vi "Autonomous Independent.vi"() -> ()   [LabVIEW 2019]
doc: "This VI is called when autonomous begins, and will automatically be terminated when autonomous ends. You can carry out timed or sensor driven robot movement independently without needing to return to the caller."
uses:
  Globals/Drive_Globals.vi
  Globals/Turret_Globals.vi
  Subsystems/Turret/Turret_States.ctl
  Subsystems/Turret/Turret_Cluster.ctl
  Globals/Flywheel_Globals.vi
  Subsystems/Flywheel/Flywheel_States.ctl
  Subsystems/Flywheel/Flywheel_Cluster.ctl
  Subsystems/Magazine/Magazine_States.ctl
  Subsystems/Magazine/Magazine_Cluster.ctl
  Globals/Magazine_Globals.vi
  Subsystems/Drive/Drive_States.ctl
  Subsystems/Drive/Drive_Cluster.ctl
  Subsystems/Intake/Intake_States.ctl
  Subsystems/Intake/Intake_Cluster.ctl
  Globals/Intake_Globals.vi
  Globals/Dash_Globals.vi
panel:
  out "Name of Play":string
  # "e"
  # "Be sure to right-click and choose Data Operations>>Make Current Value default if you want to save the array values with the VI"
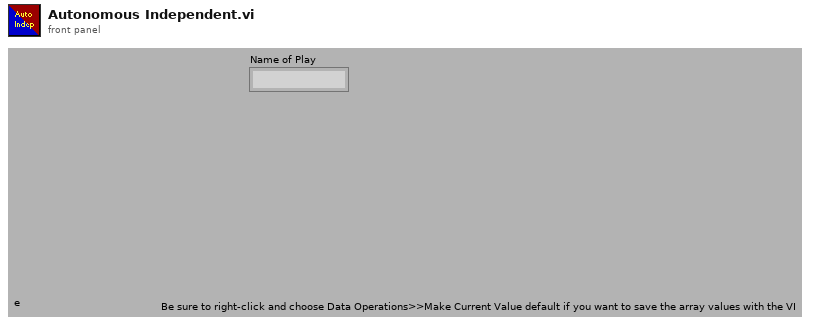
[diagram p1: front panel]
types:
  T1 = typedef "CTRE_PigeonIMU_DeviceRef.ctl" = cluster{"DeviceStatus":errorcluster, "Device Number":u8, "Type":T2, "Device ID":u32, "Handle":u64, "UsageFrame":u32, "Library Path":path}
  T2 = typedef "CTRE_PigeonIMU_ConnectionType.ctl" = u32
  T3 = typedef "WPI_MotorControlDeviceRef.ctl" = cluster{"DeviceStatus":errorcluster, "Type":T4, "PWM":cluster{"PWM Channel":T5, "DeadBand":T6}, "CAN":cluster{"Device Number":u8, "SetOutput VI Ref":variant, "GetOutput VI Ref":variant, "Enable VI Ref":variant, "Disable VI Ref":variant, "Data":variant}, "Invert":bool, "DIO PWM":cluster{"PWM \"Enable\" Channel":T5, "DIOChannel":T7, "PWM Rate":dbl}}
  T4 = typedef "WPI_MotorControlType.ctl" = enum16{"PWM", "CAN", "DIO PWM"}
  T5 = typedef "FPGA_DIOPWMChannel.ctl" = enum8{"PWM 0", "PWM 1", "PWM 2", "PWM 3", "PWM 4", "PWM 5", "PWM 6", "PWM 7", "PWM 8", "PWM 9", "PWM MXP 0", "PWM MXP 1", "PWM MXP 2", "PWM MXP 3", "PWM MXP 4", "PWM MXP 5", "PWM MXP 6", "PWM MXP 7", "PWM MXP 8", "PWM MXP 9", "Invalid"}
  T6 = typedef "WPI_PWMDeadband.ctl" = cluster{"Name":string, "maxPositivePwm":i32, "minPositivePwm":i32, "centerPwm":i32, "maxNegativePwm":i32, "minNegativePwm":i32, "angularRange":u16}
  T7 = typedef "FPGA_DIOChannel.ctl" = enum8{"DIO 0", "DIO 1", "DIO 2", "DIO 3", "DIO 4", "DIO 5", "DIO 6", "DIO 7", "DIO 8", "DIO 9", "DIO MXP 0", "DIO MXP 1", "DIO MXP 2", "DIO MXP 3", "DIO MXP 4", "DIO MXP 5", "DIO MXP 6", "DIO MXP 7", "DIO MXP 8", "DIO MXP 9", "DIO MXP 10", "DIO MXP 11", "DIO MXP 12", "DIO MXP 13", "DIO MXP 14", "DIO MXP 15", "SPI Port CS1", "SPI Port CS2", "SPI Port CS3", "SPI Port MISO", "SPI Port MOSI", "Invalid"}
  T8 = typedef "Flywheel_Cluster.ctl" = cluster{"Flywheel_Throttle":dbl, "Control_States":T9, "Auto_Speed":bool, "Flywheel_On":bool, "Parameter_1":dbl, "Parameter_2":dbl, "Auto_Notifier":refnum<notifier>, "Step":dbl}
  T9 = typedef "Flywheel_States.ctl" = enum16{"No-Op", "Percent_Voltage", "Speed_Control_Manual", "Speed_Control_Auto", "Command_SpinUp", "Command_SpinUpAuto"}
  T10 = typedef "Turret_Cluster.ctl" = cluster{"Auto-Target?":bool, "Control_State":T11, "Turret_Spin_Speed":dbl, "Turret_Spin_Speed_Control?":bool, "Step":dbl, "Parameter_1":dbl, "Parameter_2":dbl, "Parameter_3":dbl, "Auto_Notifier":refnum<notifier>, "GoToZero?":bool}
  T11 = typedef "Turret_States.ctl" = enum16{"Manual_Percent_Voltage", "Manual_Speed_Control", "Auto-Target", "Command_TurnToPosition", "Command_Auto_Target", "GoToZero"}
  T12 = typedef "Magazine_Cluster.ctl" = cluster{"Fire":bool, "Magazine_Throttle":dbl, "Control_States":T13, "Auto_Notifier":refnum<notifier>, "Parameter_1":dbl, "Parameter_2":dbl, "Step":dbl}
  T13 = typedef "Magazine_States.ctl" = enum16{"No-Op", "Loading", "Fire", "Unjam", "Manual_Percent_Voltage", "Manual_Speed_Control", "Command_Fire"}
  T14 = typedef "Drive_Cluster.ctl" = cluster{"Control_State":T15, "Angular_Throttle":dbl, "Linear_Throttle":dbl, "Torque_Changing":bool, "Step":dbl, "Parameter_1":dbl, "Parameter_2":dbl, "Parameter_3":dbl, "Parameter_4":dbl, "Auto_Notifier":refnum<notifier>}
  T15 = typedef "Drive_States.ctl" = enum16{"Percent_Voltage_Control", "Speed_Control", "Command_HeadingDistance", "Command_TurnToHeading"}
  T16 = typedef "Intake_Cluster.ctl" = cluster{"Control_State":T17, "Intake_On":bool, "Intake_Extended":bool, "Intake_Throttle":dbl, "Auto_Notifier":refnum<notifier>, "Parameter_1":dbl, "Parameter_2":dbl, "Step":dbl, "Outtake":bool}
  T17 = typedef "Intake_States.ctl" = enum16{"Manual_Control", "Compliant_Intake", "Command_RunIntake"}
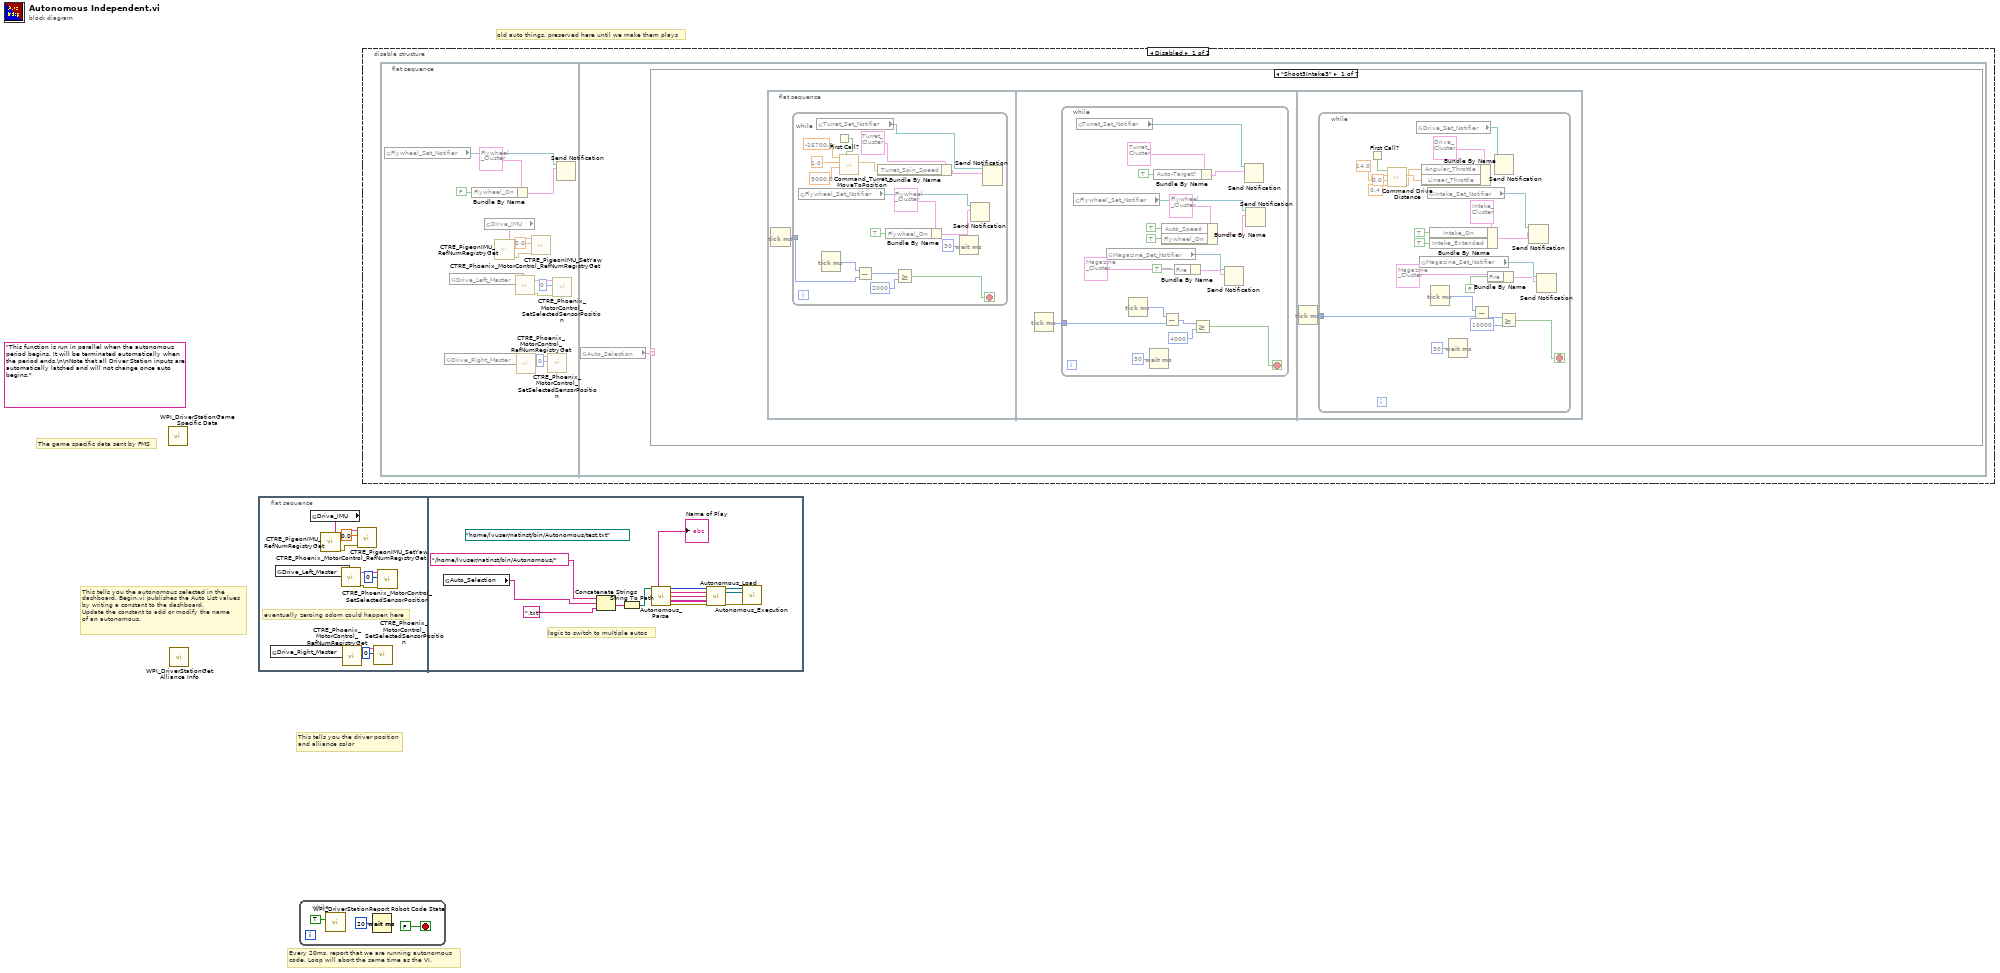
[diagram p0: block diagram]
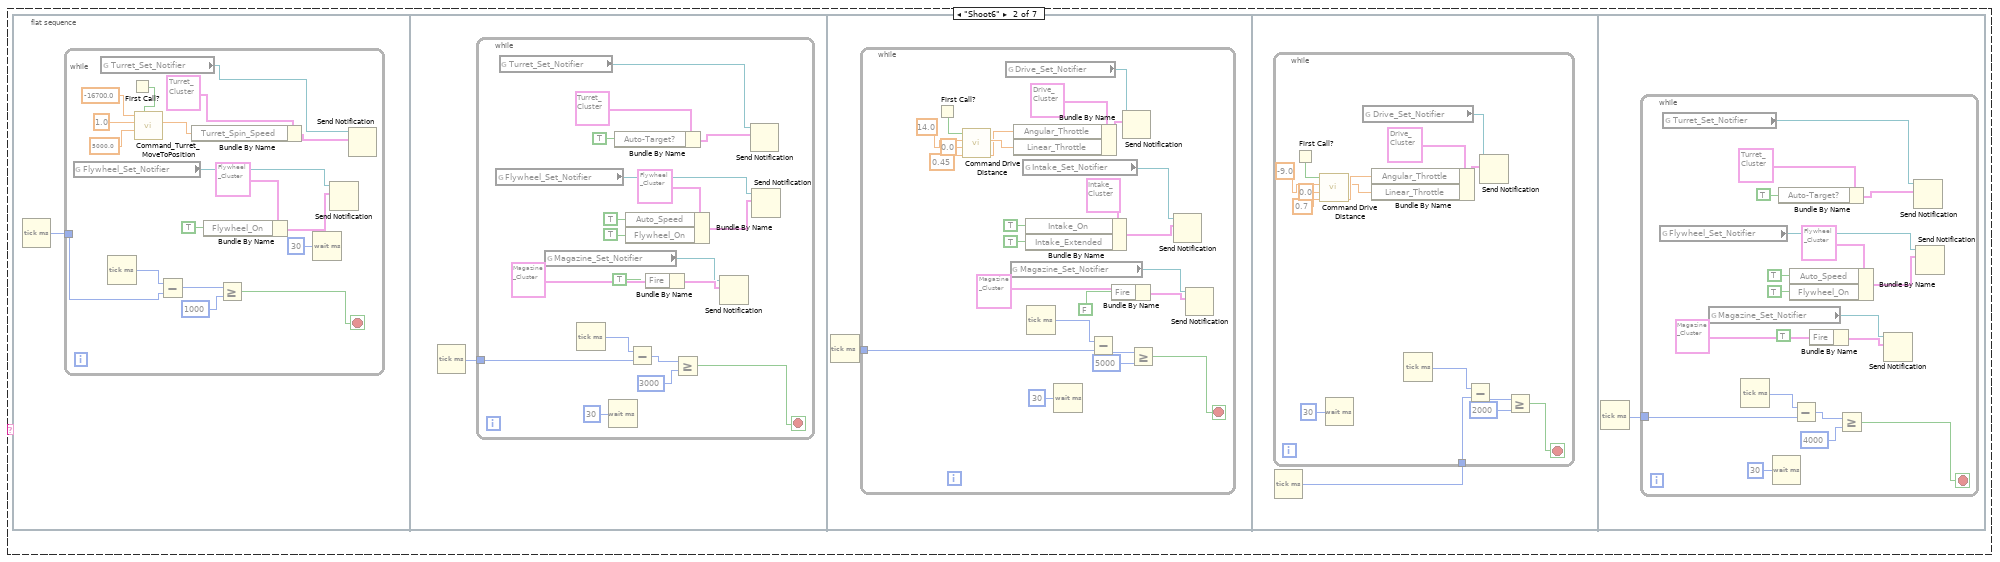
[diagram p2: hidden frame]
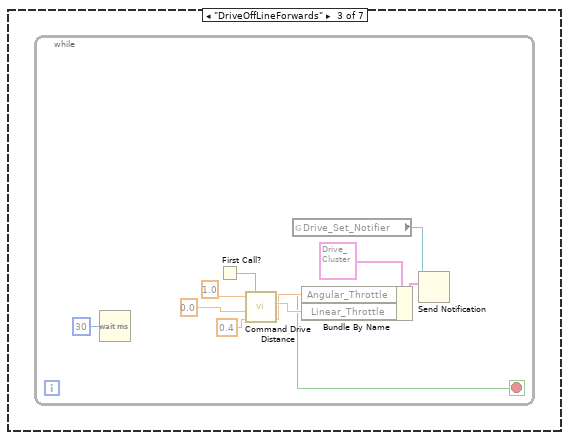
[diagram p3: hidden frame]
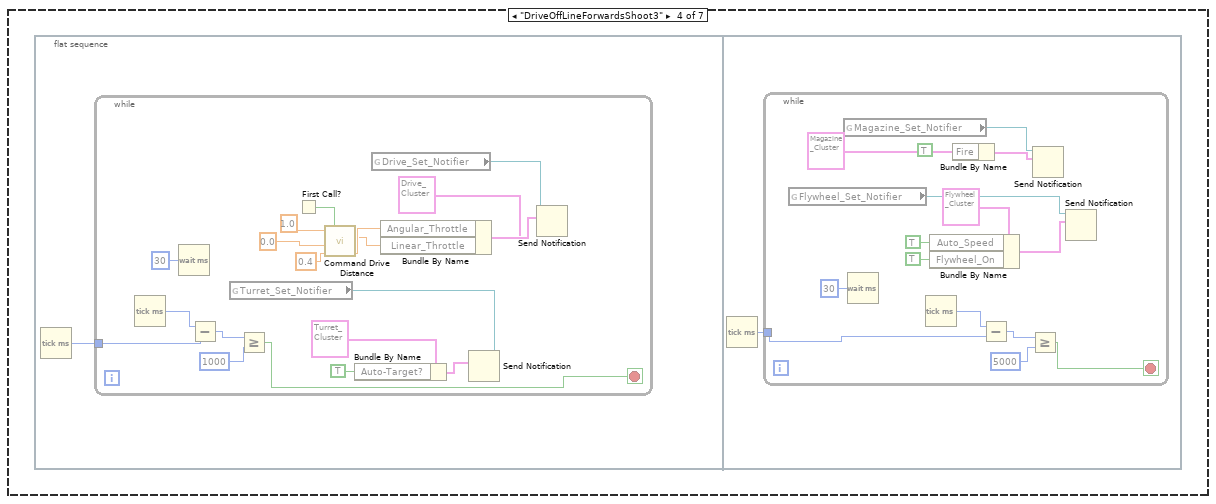
[diagram p4: hidden frame]
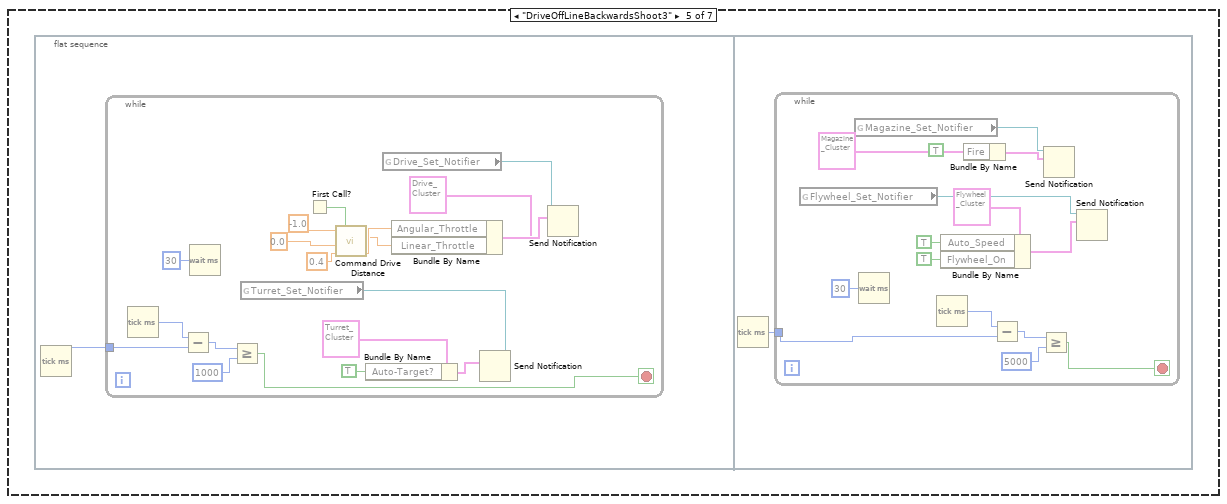
[diagram p5: hidden frame]
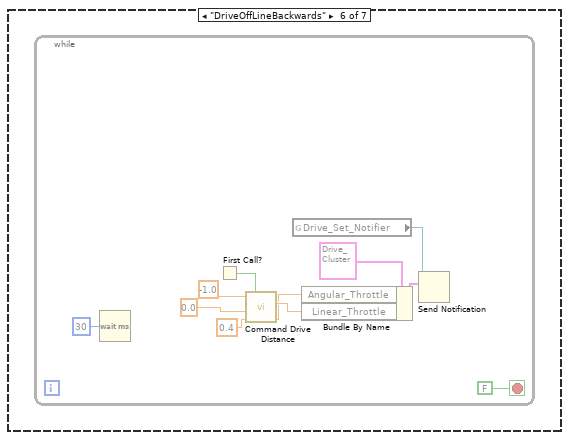
[diagram p6: hidden frame]
diagram:
  (unwired) "This function is run in parallel when the autonomous period begins. It will be terminated automatically when the period ends.\n\nNote that all Driver Station inputs are automatically latched and will not change once auto begins."
  # "old auto things, preserved here until we make them plays"
  # "The game specific data sent by FMS"
  # "This tells you the autonomous selected in the \ndashboard. Begin.vi publishes the Auto List values\nby writing a constant to the dashboard.\nUpdate the constant to add or modify the name\nof an autonomous."
  # "Every 20ms, report that we are running autonomous\ncode. Loop will abort the same time as the VI."
  # "This tells you the driver position\nand alliance color"
  n1 = call <vilib>:"WPI_DriverStationGame Specific Data.vi"() -> ()  [unwired: 11 in, 1 out]
  n2 = call <vilib>:"WPI_DriverStationGet Alliance Info.vi"() -> ()  [unwired: 12 out]
  n3 = flat-sequence {
    frame #0 {
      # "eventually zeroing odom could happen here"
      n4 = global read "Drive_Globals.vi" "Drive_Right_Master"() -> (w10:string)
      n5 = global read "Drive_Globals.vi" "Drive_Left_Master"() -> (w11:string)
      n6 = global read "Drive_Globals.vi" "Drive_IMU"() -> (w6:string)
      n7 = call <vilib>:"CTRE_PigeonIMU_RefNumRegistryGet.vi"("refnum name"=w6) -> ("error out"=w4:errorcluster, "PigeonIMUDevRef"=w5:T1)  [unwired: 9 in]
      n8 = call <vilib>:"CTRE_Phoenix_MotorControl_RefNumRegistryGet.vi"("refnum name"=w11) -> ("error out"=w8:errorcluster, "PhoenixMotorControlDevRef"=w9:T3)  [unwired: 9 in]
      n9 = call <vilib>:"CTRE_Phoenix_MotorControl_RefNumRegistryGet.vi"("refnum name"=w10) -> ("PhoenixMotorControlDevRef"=w7:T3)  [unwired: 9 in, 1 out]
      n10 = call <vilib>:"CTRE_PigeonIMU_SetYaw.vi"("error in (no error)"=w4, "Value"=0.0, "PigeonIMUDevRef"=w5) -> ()  [unwired: 7 in, 2 out]
      n11 = call <vilib>:"CTRE_Phoenix_MotorControl_SetSelectedSensorPosition.vi"("New Sensor Position"=0, "PhoenixMotorControlDevRef"=w7) -> ()  [unwired: 8 in, 2 out]
      n12 = call <vilib>:"CTRE_Phoenix_MotorControl_SetSelectedSensorPosition.vi"("error in (no error)"=w8, "New Sensor Position"=0, "PhoenixMotorControlDevRef"=w9) -> ()  [unwired: 7 in, 2 out]
    }
    frame #1 {
      (unwired) path "/home/lvuser/natinst/bin/Autonomous/test.txt" ("File Path")
      # "logic to switch to multiple autos"
      n13 = global read "Dash_Globals.vi" "Auto_Selection"() -> (w12:string)
      n14 = Concatenate Strings("/home/lvuser/natinst/bin/Autonomous/", w12, ".txt") -> (w14:string)
      n15 = String To Path(string=w14) -> (path=w13:path)
      n16 = call "Autonomous_Parse.vi"("File Path"=w13) -> ("Name of Play"=→"Name of Play":string, "Number of Commands"=w21:i32, "Subsystems"=w23:string[], "Commands"=w22:string[], "Inputs"=w25:string[][], "errror out"=w24:errorcluster)  [unwired: 8 in, 1 out]
      n17 = call "Autonomous_Load.vi"("Number of Commands"=w21, "Subsystems"=w23, "Commands"=w22, "Inputs"=w25, "error in"=w24) -> ("Queue_Key"=w19:refnum<queue>, "Autonomous_Queue"=w18:refnum<queue>, "errror out"=w20:errorcluster)  [unwired: 8 in]
      n18 = call "Autonomous_Execution.vi"("error in"=w20, "Autonomous_Queue"=w18, "Queue Key"=w19) -> ()  [unwired: 8 in, 1 out]
    }
  }
  n19 = while {
    stop <- FALSE stop-if-true
    n20 = call <vilib>:"WPI_DriverStationReport Robot Code State.vi"("Autonomous"=TRUE) -> ()  [unwired: 10 in, 1 out]
    n21 = Wait (ms)(milliseconds to wait=u32 20) -> ()  [unwired: 1 out]
  }
  n22 = disable-structure shown="Disabled" {
    frame Disabled {
      n23 = flat-sequence {
        frame #0 {
          n24 = global read "Flywheel_Globals.vi" "Flywheel_Set_Notifier"() -> (w29:refnum<notifier>)
          n25 = global read "Drive_Globals.vi" "Drive_Right_Master"() -> (w42:string)
          n26 = global read "Drive_Globals.vi" "Drive_Left_Master"() -> (w43:string)
          n27 = Bundle By Name(cluster=T8 {"Flywheel_Throttle"=0.0, "Control_States"=enum."No-Op", "Auto_Speed"=FALSE, "Flywheel_On"=FALSE, "Parameter_1"=0.0, "Parameter_2"=0.0, "Auto_Notifier"=refnum, "Step"=0.0} ("Flywheel_Cluster"), "Flywheel_On"=FALSE) -> (w30:T8)
          n28 = global read "Drive_Globals.vi" "Drive_IMU"() -> (w38:string)
          n29 = call <vilib>:"CTRE_PigeonIMU_RefNumRegistryGet.vi"("refnum name"=w38) -> ("error out"=w36:errorcluster, "PigeonIMUDevRef"=w37:T1)  [unwired: 9 in]
          n30 = call <vilib>:"CTRE_Phoenix_MotorControl_RefNumRegistryGet.vi"("refnum name"=w43) -> ("error out"=w40:errorcluster, "PhoenixMotorControlDevRef"=w41:T3)  [unwired: 9 in]
          n31 = call <vilib>:"CTRE_Phoenix_MotorControl_RefNumRegistryGet.vi"("refnum name"=w42) -> ("PhoenixMotorControlDevRef"=w39:T3)  [unwired: 9 in, 1 out]
          n32 = call <vilib>:"CTRE_PigeonIMU_SetYaw.vi"("error in (no error)"=w36, "Value"=0.0, "PigeonIMUDevRef"=w37) -> ()  [unwired: 7 in, 2 out]
          n33 = call <vilib>:"CTRE_Phoenix_MotorControl_SetSelectedSensorPosition.vi"("New Sensor Position"=0, "PhoenixMotorControlDevRef"=w39) -> ()  [unwired: 8 in, 2 out]
          n34 = call <vilib>:"CTRE_Phoenix_MotorControl_SetSelectedSensorPosition.vi"("error in (no error)"=w40, "New Sensor Position"=0, "PhoenixMotorControlDevRef"=w41) -> ()  [unwired: 7 in, 2 out]
          n35 = Send Notification(notification=w30, notifier=w29) -> ()  [unwired: 1 in, 2 out]
        }
        frame #1 {
          n36 = global read "Dash_Globals.vi" "Auto_Selection"() -> (w44:string)
          n37 = case shown="\"Shoot3Intake3\"" w44 {
            frame "Shoot3Intake3" {
              n38 = flat-sequence {
                frame #0 {
                  n39 = Tick Count (ms)() -> (millisecond timer value=w45:u32)
                  n40 = while {
                    tunnel: w45 -> [w53]
                    stop <- w50 stop-if-true
                    n41 = global read "Flywheel_Globals.vi" "Flywheel_Set_Notifier"() -> (w49:refnum<notifier>)
                    n42 = global read "Turret_Globals.vi" "Turret_Set_Notifier"() -> (w59:refnum<notifier>)
                    n43 = Tick Count (ms)() -> (millisecond timer value=w54:u32)
                    n44 = First Call?() -> (First Call?: T/F=w60:bool)
                    n45 = call "Command_Turret_MoveToPosition.vi"("Startup"=w60, "Timeout"=5000.0, "Speed"=1.0, "Goal_Position"=-16700.0) -> ("Turret_Speed"=w56:dbl)  [unwired: 5 in, 2 out]
                    n46 = Subtract(x=w54, y=w53) -> (x-y=w51:u32)
                    n47 = Bundle By Name(cluster=T10 {"Auto-Target?"=FALSE, "Control_State"=enum."Manual_Percent_Voltage", "Turret_Spin_Speed"=0.0, "Turret_Spin_Speed_Control?"=FALSE, "Step"=0.0, "Parameter_1"=0.0, "Parameter_2"=0.0, "Parameter_3"=0.0, "Auto_Notifier"=refnum, "GoToZero?"=FALSE} ("Turret_Cluster"), "Turret_Spin_Speed"=w56) -> (w57:T10)
                    n48 = Bundle By Name(cluster=T8 {"Flywheel_Throttle"=0.0, "Control_States"=enum."No-Op", "Auto_Speed"=FALSE, "Flywheel_On"=FALSE, "Parameter_1"=0.0, "Parameter_2"=0.0, "Auto_Notifier"=refnum, "Step"=0.0} ("Flywheel_Cluster"), "Flywheel_On"=TRUE) -> (w48:T8)
                    n49 = Greater Or Equal?(x=w51, y=u32 2000) -> (x >= y?=w50:bool)
                    n50 = Wait (ms)(milliseconds to wait=u32 30) -> ()  [unwired: 1 out]
                    n51 = Send Notification(notification=w48, notifier=w49) -> ()  [unwired: 1 in, 2 out]
                    n52 = Send Notification(notification=w57, notifier=w59) -> ()  [unwired: 1 in, 2 out]
                  }
                }
                frame #1 {
                  n53 = Tick Count (ms)() -> (millisecond timer value=w64:u32)
                  n54 = while {
                    tunnel: w64 -> [w68]
                    stop <- w65 stop-if-true
                    n55 = global read "Flywheel_Globals.vi" "Flywheel_Set_Notifier"() -> (w79:refnum<notifier>)
                    n56 = global read "Turret_Globals.vi" "Turret_Set_Notifier"() -> (w83:refnum<notifier>)
                    n57 = global read "Magazine_Globals.vi" "Magazine_Set_Notifier"() -> (w71:refnum<notifier>)
                    n58 = Tick Count (ms)() -> (millisecond timer value=w69:u32)
                    n59 = Wait (ms)(milliseconds to wait=u32 30) -> ()  [unwired: 1 out]
                    n60 = Bundle By Name(cluster=T10 {"Auto-Target?"=FALSE, "Control_State"=enum."Manual_Percent_Voltage", "Turret_Spin_Speed"=0.0, "Turret_Spin_Speed_Control?"=FALSE, "Step"=0.0, "Parameter_1"=0.0, "Parameter_2"=0.0, "Parameter_3"=0.0, "Auto_Notifier"=refnum, "GoToZero?"=FALSE} ("Turret_Cluster"), "Auto-Target?"=TRUE) -> (w81:T10)
                    n61 = Bundle By Name(cluster=T8 {"Flywheel_Throttle"=0.0, "Control_States"=enum."No-Op", "Auto_Speed"=FALSE, "Flywheel_On"=FALSE, "Parameter_1"=0.0, "Parameter_2"=0.0, "Auto_Notifier"=refnum, "Step"=0.0} ("Flywheel_Cluster"), "Auto_Speed"=TRUE, "Flywheel_On"=TRUE) -> (w78:T8)
                    n62 = Subtract(x=w69, y=w68) -> (x-y=w67:u32)
                    n63 = Bundle By Name(cluster=T12 {"Fire"=FALSE, "Magazine_Throttle"=0.0, "Control_States"=enum."No-Op", "Auto_Notifier"=refnum, "Parameter_1"=0.0, "Parameter_2"=0.0, "Step"=0.0} ("Magazine_Cluster"), "Fire"=TRUE) -> (w72:T12)
                    n64 = Greater Or Equal?(x=w67, y=u32 4000) -> (x >= y?=w65:bool)
                    n65 = Send Notification(notification=w72, notifier=w71) -> ()  [unwired: 1 in, 2 out]
                    n66 = Send Notification(notification=w81, notifier=w83) -> ()  [unwired: 1 in, 2 out]
                    n67 = Send Notification(notification=w78, notifier=w79) -> ()  [unwired: 1 in, 2 out]
                  }
                }
                frame #2 {
                  n68 = Tick Count (ms)() -> (millisecond timer value=w84:u32)
                  n69 = while {
                    tunnel: w84 -> [w107]
                    stop <- w98 stop-if-true
                    n70 = First Call?() -> (First Call?: T/F=w94:bool)
                    n71 = call "Command Drive Distance.vi"("Speed"=0.4, "Heading"=0.0, "Distance(Feet)"=14.0 ("Distance"), "Startup"=w94) -> ("Angular"=w95:dbl, "Linear"=w96:dbl)  [unwired: 4 in, 2 out]
                    n72 = global read "Drive_Globals.vi" "Drive_Set_Notifier"() -> (w93:refnum<notifier>)
                    n73 = global read "Magazine_Globals.vi" "Magazine_Set_Notifier"() -> (w88:refnum<notifier>)
                    n74 = Bundle By Name(cluster=T14 {"Control_State"=enum."Percent_Voltage_Control", "Angular_Throttle"=0.0, "Linear_Throttle"=0.0, "Torque_Changing"=FALSE, "Step"=0.0, "Parameter_1"=0.0, "Parameter_2"=0.0, "Parameter_3"=0.0, "Parameter_4"=0.0, "Auto_Notifier"=refnum} ("Drive_Cluster"), "Angular_Throttle"=w95, "Linear_Throttle"=w96) -> (w97:T14)
                    n75 = global read "Intake_Globals.vi" "Intake_Set_Notifier"() -> (w102:refnum<notifier>)
                    n76 = Bundle By Name(cluster=T16 {"Control_State"=enum."Manual_Control", "Intake_On"=FALSE, "Intake_Extended"=FALSE, "Intake_Throttle"=0.0, "Auto_Notifier"=refnum, "Parameter_1"=0.0, "Parameter_2"=0.0, "Step"=0.0, "Outtake"=FALSE} ("Intake_Cluster"), "Intake_On"=TRUE ("Intake"), "Intake_Extended"=TRUE) -> (w101:T16)
                    n77 = Tick Count (ms)() -> (millisecond timer value=w108:u32)
                    n78 = Wait (ms)(milliseconds to wait=u32 30) -> ()  [unwired: 1 out]
                    n79 = Subtract(x=w108, y=w107) -> (x-y=w105:u32)
                    n80 = Bundle By Name(cluster=T12 {"Fire"=FALSE, "Magazine_Throttle"=0.0, "Control_States"=enum."No-Op", "Auto_Notifier"=refnum, "Parameter_1"=0.0, "Parameter_2"=0.0, "Step"=0.0} ("Magazine_Cluster"), "Fire"=FALSE) -> (w87:T12)
                    n81 = Send Notification(notification=w97, notifier=w93) -> ()  [unwired: 1 in, 2 out]
                    n82 = Greater Or Equal?(x=w105, y=u32 10000) -> (x >= y?=w98:bool)
                    n83 = Send Notification(notification=w101, notifier=w102) -> ()  [unwired: 1 in, 2 out]
                    n84 = Send Notification(notification=w87, notifier=w88) -> ()  [unwired: 1 in, 2 out]
                  }
                }
              }
            }
            frame "Shoot6" {
              n85 = flat-sequence {
                frame #0 {
                  n86 = Tick Count (ms)() -> (millisecond timer value=w109:u32)
                  n87 = while {
                    tunnel: w109 -> [w117]
                    stop <- w114 stop-if-true
                    n88 = global read "Flywheel_Globals.vi" "Flywheel_Set_Notifier"() -> (w113:refnum<notifier>)
                    n89 = global read "Turret_Globals.vi" "Turret_Set_Notifier"() -> (w123:refnum<notifier>)
                    n90 = Tick Count (ms)() -> (millisecond timer value=w118:u32)
                    n91 = First Call?() -> (First Call?: T/F=w124:bool)
                    n92 = call "Command_Turret_MoveToPosition.vi"("Startup"=w124, "Timeout"=5000.0, "Speed"=1.0, "Goal_Position"=-16700.0) -> ("Turret_Speed"=w120:dbl)  [unwired: 5 in, 2 out]
                    n93 = Subtract(x=w118, y=w117) -> (x-y=w115:u32)
                    n94 = Bundle By Name(cluster=T10 {"Auto-Target?"=FALSE, "Control_State"=enum."Manual_Percent_Voltage", "Turret_Spin_Speed"=0.0, "Turret_Spin_Speed_Control?"=FALSE, "Step"=0.0, "Parameter_1"=0.0, "Parameter_2"=0.0, "Parameter_3"=0.0, "Auto_Notifier"=refnum, "GoToZero?"=FALSE} ("Turret_Cluster"), "Turret_Spin_Speed"=w120) -> (w121:T10)
                    n95 = Bundle By Name(cluster=T8 {"Flywheel_Throttle"=0.0, "Control_States"=enum."No-Op", "Auto_Speed"=FALSE, "Flywheel_On"=FALSE, "Parameter_1"=0.0, "Parameter_2"=0.0, "Auto_Notifier"=refnum, "Step"=0.0} ("Flywheel_Cluster"), "Flywheel_On"=TRUE) -> (w112:T8)
                    n96 = Greater Or Equal?(x=w115, y=u32 1000) -> (x >= y?=w114:bool)
                    n97 = Wait (ms)(milliseconds to wait=u32 30) -> ()  [unwired: 1 out]
                    n98 = Send Notification(notification=w112, notifier=w113) -> ()  [unwired: 1 in, 2 out]
                    n99 = Send Notification(notification=w121, notifier=w123) -> ()  [unwired: 1 in, 2 out]
                  }
                }
                frame #1 {
                  n100 = Tick Count (ms)() -> (millisecond timer value=w128:u32)
                  n101 = while {
                    tunnel: w128 -> [w132]
                    stop <- w129 stop-if-true
                    n102 = global read "Flywheel_Globals.vi" "Flywheel_Set_Notifier"() -> (w143:refnum<notifier>)
                    n103 = global read "Turret_Globals.vi" "Turret_Set_Notifier"() -> (w147:refnum<notifier>)
                    n104 = global read "Magazine_Globals.vi" "Magazine_Set_Notifier"() -> (w135:refnum<notifier>)
                    n105 = Tick Count (ms)() -> (millisecond timer value=w133:u32)
                    n106 = Wait (ms)(milliseconds to wait=u32 30) -> ()  [unwired: 1 out]
                    n107 = Bundle By Name(cluster=T10 {"Auto-Target?"=FALSE, "Control_State"=enum."Manual_Percent_Voltage", "Turret_Spin_Speed"=0.0, "Turret_Spin_Speed_Control?"=FALSE, "Step"=0.0, "Parameter_1"=0.0, "Parameter_2"=0.0, "Parameter_3"=0.0, "Auto_Notifier"=refnum, "GoToZero?"=FALSE} ("Turret_Cluster"), "Auto-Target?"=TRUE) -> (w145:T10)
                    n108 = Bundle By Name(cluster=T8 {"Flywheel_Throttle"=0.0, "Control_States"=enum."No-Op", "Auto_Speed"=FALSE, "Flywheel_On"=FALSE, "Parameter_1"=0.0, "Parameter_2"=0.0, "Auto_Notifier"=refnum, "Step"=0.0} ("Flywheel_Cluster"), "Auto_Speed"=TRUE, "Flywheel_On"=TRUE) -> (w142:T8)
                    n109 = Subtract(x=w133, y=w132) -> (x-y=w131:u32)
                    n110 = Bundle By Name(cluster=T12 {"Fire"=FALSE, "Magazine_Throttle"=0.0, "Control_States"=enum."No-Op", "Auto_Notifier"=refnum, "Parameter_1"=0.0, "Parameter_2"=0.0, "Step"=0.0} ("Magazine_Cluster"), "Fire"=TRUE) -> (w136:T12)
                    n111 = Greater Or Equal?(x=w131, y=u32 3000) -> (x >= y?=w129:bool)
                    n112 = Send Notification(notification=w136, notifier=w135) -> ()  [unwired: 1 in, 2 out]
                    n113 = Send Notification(notification=w145, notifier=w147) -> ()  [unwired: 1 in, 2 out]
                    n114 = Send Notification(notification=w142, notifier=w143) -> ()  [unwired: 1 in, 2 out]
                  }
                }
                frame #2 {
                  n115 = Tick Count (ms)() -> (millisecond timer value=w148:u32)
                  n116 = while {
                    tunnel: w148 -> [w171]
                    stop <- w162 stop-if-true
                    n117 = First Call?() -> (First Call?: T/F=w158:bool)
                    n118 = call "Command Drive Distance.vi"("Speed"=0.45, "Heading"=0.0, "Distance(Feet)"=14.0 ("Distance"), "Startup"=w158) -> ("Angular"=w159:dbl, "Linear"=w160:dbl)  [unwired: 4 in, 2 out]
                    n119 = global read "Drive_Globals.vi" "Drive_Set_Notifier"() -> (w157:refnum<notifier>)
                    n120 = global read "Magazine_Globals.vi" "Magazine_Set_Notifier"() -> (w152:refnum<notifier>)
                    n121 = Bundle By Name(cluster=T14 {"Control_State"=enum."Percent_Voltage_Control", "Angular_Throttle"=0.0, "Linear_Throttle"=0.0, "Torque_Changing"=FALSE, "Step"=0.0, "Parameter_1"=0.0, "Parameter_2"=0.0, "Parameter_3"=0.0, "Parameter_4"=0.0, "Auto_Notifier"=refnum} ("Drive_Cluster"), "Angular_Throttle"=w159, "Linear_Throttle"=w160) -> (w161:T14)
                    n122 = global read "Intake_Globals.vi" "Intake_Set_Notifier"() -> (w166:refnum<notifier>)
                    n123 = Bundle By Name(cluster=T16 {"Control_State"=enum."Manual_Control", "Intake_On"=FALSE, "Intake_Extended"=FALSE, "Intake_Throttle"=0.0, "Auto_Notifier"=refnum, "Parameter_1"=0.0, "Parameter_2"=0.0, "Step"=0.0, "Outtake"=FALSE} ("Intake_Cluster"), "Intake_On"=TRUE ("Intake"), "Intake_Extended"=TRUE) -> (w165:T16)
                    n124 = Tick Count (ms)() -> (millisecond timer value=w172:u32)
                    n125 = Wait (ms)(milliseconds to wait=u32 30) -> ()  [unwired: 1 out]
                    n126 = Subtract(x=w172, y=w171) -> (x-y=w169:u32)
                    n127 = Bundle By Name(cluster=T12 {"Fire"=FALSE, "Magazine_Throttle"=0.0, "Control_States"=enum."No-Op", "Auto_Notifier"=refnum, "Parameter_1"=0.0, "Parameter_2"=0.0, "Step"=0.0} ("Magazine_Cluster"), "Fire"=FALSE) -> (w151:T12)
                    n128 = Send Notification(notification=w161, notifier=w157) -> ()  [unwired: 1 in, 2 out]
                    n129 = Greater Or Equal?(x=w169, y=u32 5000) -> (x >= y?=w162:bool)
                    n130 = Send Notification(notification=w165, notifier=w166) -> ()  [unwired: 1 in, 2 out]
                    n131 = Send Notification(notification=w151, notifier=w152) -> ()  [unwired: 1 in, 2 out]
                  }
                }
                frame #3 {
                  n132 = Tick Count (ms)() -> (millisecond timer value=w173:u32)
                  n133 = while {
                    tunnel: w173 -> [w176]
                    stop <- w175 stop-if-true
                    n134 = First Call?() -> (First Call?: T/F=w184:bool)
                    n135 = call "Command Drive Distance.vi"("Speed"=0.7, "Heading"=0.0, "Distance(Feet)"=-9.0 ("Distance"), "Startup"=w184) -> ("Angular"=w183:dbl, "Linear"=w182:dbl)  [unwired: 4 in, 2 out]
                    n136 = Wait (ms)(milliseconds to wait=u32 30) -> ()  [unwired: 1 out]
                    n137 = global read "Drive_Globals.vi" "Drive_Set_Notifier"() -> (w185:refnum<notifier>)
                    n138 = Bundle By Name(cluster=T14 {"Control_State"=enum."Percent_Voltage_Control", "Angular_Throttle"=0.0, "Linear_Throttle"=0.0, "Torque_Changing"=FALSE, "Step"=0.0, "Parameter_1"=0.0, "Parameter_2"=0.0, "Parameter_3"=0.0, "Parameter_4"=0.0, "Auto_Notifier"=refnum} ("Drive_Cluster"), "Angular_Throttle"=w183, "Linear_Throttle"=w182) -> (w181:T14)
                    n139 = Tick Count (ms)() -> (millisecond timer value=w177:u32)
                    n140 = Subtract(x=w177, y=w176) -> (x-y=w178:u32)
                    n141 = Send Notification(notification=w181, notifier=w185) -> ()  [unwired: 1 in, 2 out]
                    n142 = Greater Or Equal?(x=w178, y=u32 2000) -> (x >= y?=w175:bool)
                  }
                }
                frame #4 {
                  n143 = Tick Count (ms)() -> (millisecond timer value=w189:u32)
                  n144 = while {
                    tunnel: w189 -> [w193]
                    stop <- w190 stop-if-true
                    n145 = global read "Flywheel_Globals.vi" "Flywheel_Set_Notifier"() -> (w204:refnum<notifier>)
                    n146 = global read "Turret_Globals.vi" "Turret_Set_Notifier"() -> (w208:refnum<notifier>)
                    n147 = global read "Magazine_Globals.vi" "Magazine_Set_Notifier"() -> (w196:refnum<notifier>)
                    n148 = Tick Count (ms)() -> (millisecond timer value=w194:u32)
                    n149 = Wait (ms)(milliseconds to wait=u32 30) -> ()  [unwired: 1 out]
                    n150 = Bundle By Name(cluster=T10 {"Auto-Target?"=FALSE, "Control_State"=enum."Manual_Percent_Voltage", "Turret_Spin_Speed"=0.0, "Turret_Spin_Speed_Control?"=FALSE, "Step"=0.0, "Parameter_1"=0.0, "Parameter_2"=0.0, "Parameter_3"=0.0, "Auto_Notifier"=refnum, "GoToZero?"=FALSE} ("Turret_Cluster"), "Auto-Target?"=TRUE) -> (w206:T10)
                    n151 = Bundle By Name(cluster=T8 {"Flywheel_Throttle"=0.0, "Control_States"=enum."No-Op", "Auto_Speed"=FALSE, "Flywheel_On"=FALSE, "Parameter_1"=0.0, "Parameter_2"=0.0, "Auto_Notifier"=refnum, "Step"=0.0} ("Flywheel_Cluster"), "Auto_Speed"=TRUE, "Flywheel_On"=TRUE) -> (w203:T8)
                    n152 = Subtract(x=w194, y=w193) -> (x-y=w192:u32)
                    n153 = Bundle By Name(cluster=T12 {"Fire"=FALSE, "Magazine_Throttle"=0.0, "Control_States"=enum."No-Op", "Auto_Notifier"=refnum, "Parameter_1"=0.0, "Parameter_2"=0.0, "Step"=0.0} ("Magazine_Cluster"), "Fire"=TRUE) -> (w197:T12)
                    n154 = Greater Or Equal?(x=w192, y=u32 4000) -> (x >= y?=w190:bool)
                    n155 = Send Notification(notification=w197, notifier=w196) -> ()  [unwired: 1 in, 2 out]
                    n156 = Send Notification(notification=w206, notifier=w208) -> ()  [unwired: 1 in, 2 out]
                    n157 = Send Notification(notification=w203, notifier=w204) -> ()  [unwired: 1 in, 2 out]
                  }
                }
              }
            }
            frame "DriveOffLineForwards" {
              n158 = while {
                stop <- w209 stop-if-true
                n159 = Wait (ms)(milliseconds to wait=u32 30) -> ()  [unwired: 1 out]
                n160 = First Call?() -> (First Call?: T/F=w216:bool)
                n161 = call "Command Drive Distance.vi"("Speed"=0.4, "Heading"=0.0, "Distance(Feet)"=1.0 ("Distance"), "Startup"=w216) -> ("Angular"=w217:dbl, "Linear"=w218:dbl, "Completed"=w209:bool)  [unwired: 4 in, 1 out]
                n162 = global read "Drive_Globals.vi" "Drive_Set_Notifier"() -> (w215:refnum<notifier>)
                n163 = Bundle By Name(cluster=T14 {"Control_State"=enum."Percent_Voltage_Control", "Angular_Throttle"=0.0, "Linear_Throttle"=0.0, "Torque_Changing"=FALSE, "Step"=0.0, "Parameter_1"=0.0, "Parameter_2"=0.0, "Parameter_3"=0.0, "Parameter_4"=0.0, "Auto_Notifier"=refnum} ("Drive_Cluster"), "Angular_Throttle"=w217, "Linear_Throttle"=w218) -> (w219:T14)
                n164 = Send Notification(notification=w219, notifier=w215) -> ()  [unwired: 1 in, 2 out]
              }
            }
            frame "DriveOffLineForwardsShoot3" {
              n165 = flat-sequence {
                frame #0 {
                  n166 = Tick Count (ms)() -> (millisecond timer value=w220:u32)
                  n167 = while {
                    tunnel: w220 -> [w222]
                    stop <- w221 stop-if-true
                    n168 = Tick Count (ms)() -> (millisecond timer value=w224:u32)
                    n169 = Wait (ms)(milliseconds to wait=u32 30) -> ()  [unwired: 1 out]
                    n170 = Subtract(x=w224, y=w222) -> (x-y=w225:u32)
                    n171 = global read "Turret_Globals.vi" "Turret_Set_Notifier"() -> (w231:refnum<notifier>)
                    n172 = Greater Or Equal?(x=w225, y=u32 1000) -> (x >= y?=w221:bool)
                    n173 = First Call?() -> (First Call?: T/F=w226:bool)
                    n174 = call "Command Drive Distance.vi"("Speed"=0.4, "Heading"=0.0, "Distance(Feet)"=1.0 ("Distance"), "Startup"=w226) -> ("Angular"=w238:dbl, "Linear"=w227:dbl)  [unwired: 4 in, 2 out]
                    n175 = Bundle By Name(cluster=T10 {"Auto-Target?"=FALSE, "Control_State"=enum."Manual_Percent_Voltage", "Turret_Spin_Speed"=0.0, "Turret_Spin_Speed_Control?"=FALSE, "Step"=0.0, "Parameter_1"=0.0, "Parameter_2"=0.0, "Parameter_3"=0.0, "Auto_Notifier"=refnum, "GoToZero?"=FALSE} ("Turret_Cluster"), "Auto-Target?"=TRUE) -> (w229:T10)
                    n176 = global read "Drive_Globals.vi" "Drive_Set_Notifier"() -> (w237:refnum<notifier>)
                    n177 = Bundle By Name(cluster=T14 {"Control_State"=enum."Percent_Voltage_Control", "Angular_Throttle"=0.0, "Linear_Throttle"=0.0, "Torque_Changing"=FALSE, "Step"=0.0, "Parameter_1"=0.0, "Parameter_2"=0.0, "Parameter_3"=0.0, "Parameter_4"=0.0, "Auto_Notifier"=refnum} ("Drive_Cluster"), "Angular_Throttle"=w238, "Linear_Throttle"=w227) -> (w239:T14)
                    n178 = Send Notification(notification=w229, notifier=w231) -> ()  [unwired: 1 in, 2 out]
                    n179 = Send Notification(notification=w239, notifier=w237) -> ()  [unwired: 1 in, 2 out]
                  }
                }
                frame #1 {
                  n180 = Tick Count (ms)() -> (millisecond timer value=w240:u32)
                  n181 = while {
                    tunnel: w240 -> [w241]
                    stop <- w246 stop-if-true
                    n182 = global read "Flywheel_Globals.vi" "Flywheel_Set_Notifier"() -> (w255:refnum<notifier>)
                    n183 = global read "Magazine_Globals.vi" "Magazine_Set_Notifier"() -> (w242:refnum<notifier>)
                    n184 = Wait (ms)(milliseconds to wait=u32 30) -> ()  [unwired: 1 out]
                    n185 = Tick Count (ms)() -> (millisecond timer value=w249:u32)
                    n186 = Bundle By Name(cluster=T8 {"Flywheel_Throttle"=0.0, "Control_States"=enum."No-Op", "Auto_Speed"=FALSE, "Flywheel_On"=FALSE, "Parameter_1"=0.0, "Parameter_2"=0.0, "Auto_Notifier"=refnum, "Step"=0.0} ("Flywheel_Cluster"), "Auto_Speed"=TRUE, "Flywheel_On"=TRUE) -> (w254:T8)
                    n187 = Bundle By Name(cluster=T12 {"Fire"=FALSE, "Magazine_Throttle"=0.0, "Control_States"=enum."No-Op", "Auto_Notifier"=refnum, "Parameter_1"=0.0, "Parameter_2"=0.0, "Step"=0.0} ("Magazine_Cluster"), "Fire"=TRUE) -> (w243:T12)
                    n188 = Subtract(x=w249, y=w241) -> (x-y=w248:u32)
                    n189 = Greater Or Equal?(x=w248, y=u32 5000) -> (x >= y?=w246:bool)
                    n190 = Send Notification(notification=w243, notifier=w242) -> ()  [unwired: 1 in, 2 out]
                    n191 = Send Notification(notification=w254, notifier=w255) -> ()  [unwired: 1 in, 2 out]
                  }
                }
              }
            }
            frame "DriveOffLineBackwardsShoot3" {
              n192 = flat-sequence {
                frame #0 {
                  n193 = Tick Count (ms)() -> (millisecond timer value=w256:u32)
                  n194 = while {
                    tunnel: w256 -> [w258]
                    stop <- w257 stop-if-true
                    n195 = Tick Count (ms)() -> (millisecond timer value=w259:u32)
                    n196 = Subtract(x=w259, y=w258) -> (x-y=w260:u32)
                    n197 = Wait (ms)(milliseconds to wait=u32 30) -> ()  [unwired: 1 out]
                    n198 = Greater Or Equal?(x=w260, y=u32 1000) -> (x >= y?=w257:bool)
                    n199 = global read "Turret_Globals.vi" "Turret_Set_Notifier"() -> (w267:refnum<notifier>)
                    n200 = First Call?() -> (First Call?: T/F=w262:bool)
                    n201 = call "Command Drive Distance.vi"("Speed"=0.4, "Heading"=0.0, "Distance(Feet)"=-1.0 ("Distance"), "Startup"=w262) -> ("Angular"=w274:dbl, "Linear"=w263:dbl)  [unwired: 4 in, 2 out]
                    n202 = Bundle By Name(cluster=T10 {"Auto-Target?"=FALSE, "Control_State"=enum."Manual_Percent_Voltage", "Turret_Spin_Speed"=0.0, "Turret_Spin_Speed_Control?"=FALSE, "Step"=0.0, "Parameter_1"=0.0, "Parameter_2"=0.0, "Parameter_3"=0.0, "Auto_Notifier"=refnum, "GoToZero?"=FALSE} ("Turret_Cluster"), "Auto-Target?"=TRUE) -> (w265:T10)
                    n203 = global read "Drive_Globals.vi" "Drive_Set_Notifier"() -> (w273:refnum<notifier>)
                    n204 = Bundle By Name(cluster=T14 {"Control_State"=enum."Percent_Voltage_Control", "Angular_Throttle"=0.0, "Linear_Throttle"=0.0, "Torque_Changing"=FALSE, "Step"=0.0, "Parameter_1"=0.0, "Parameter_2"=0.0, "Parameter_3"=0.0, "Parameter_4"=0.0, "Auto_Notifier"=refnum} ("Drive_Cluster"), "Angular_Throttle"=w274, "Linear_Throttle"=w263) -> (w275:T14)
                    n205 = Send Notification(notification=w265, notifier=w267) -> ()  [unwired: 1 in, 2 out]
                    n206 = Send Notification(notification=w275, notifier=w273) -> ()  [unwired: 1 in, 2 out]
                  }
                }
                frame #1 {
                  n207 = Tick Count (ms)() -> (millisecond timer value=w276:u32)
                  n208 = while {
                    tunnel: w276 -> [w277]
                    stop <- w282 stop-if-true
                    n209 = global read "Flywheel_Globals.vi" "Flywheel_Set_Notifier"() -> (w291:refnum<notifier>)
                    n210 = global read "Magazine_Globals.vi" "Magazine_Set_Notifier"() -> (w278:refnum<notifier>)
                    n211 = Wait (ms)(milliseconds to wait=u32 30) -> ()  [unwired: 1 out]
                    n212 = Tick Count (ms)() -> (millisecond timer value=w285:u32)
                    n213 = Bundle By Name(cluster=T8 {"Flywheel_Throttle"=0.0, "Control_States"=enum."No-Op", "Auto_Speed"=FALSE, "Flywheel_On"=FALSE, "Parameter_1"=0.0, "Parameter_2"=0.0, "Auto_Notifier"=refnum, "Step"=0.0} ("Flywheel_Cluster"), "Auto_Speed"=TRUE, "Flywheel_On"=TRUE) -> (w290:T8)
                    n214 = Bundle By Name(cluster=T12 {"Fire"=FALSE, "Magazine_Throttle"=0.0, "Control_States"=enum."No-Op", "Auto_Notifier"=refnum, "Parameter_1"=0.0, "Parameter_2"=0.0, "Step"=0.0} ("Magazine_Cluster"), "Fire"=TRUE) -> (w279:T12)
                    n215 = Subtract(x=w285, y=w277) -> (x-y=w284:u32)
                    n216 = Greater Or Equal?(x=w284, y=u32 5000) -> (x >= y?=w282:bool)
                    n217 = Send Notification(notification=w279, notifier=w278) -> ()  [unwired: 1 in, 2 out]
                    n218 = Send Notification(notification=w290, notifier=w291) -> ()  [unwired: 1 in, 2 out]
                  }
                }
              }
            }
            frame "DriveOffLineBackwards" {
              n219 = while {
                stop <- FALSE stop-if-true
                n220 = Wait (ms)(milliseconds to wait=u32 30) -> ()  [unwired: 1 out]
                n221 = First Call?() -> (First Call?: T/F=w299:bool)
                n222 = call "Command Drive Distance.vi"("Speed"=0.4, "Heading"=0.0, "Distance(Feet)"=-1.0 ("Distance"), "Startup"=w299) -> ("Angular"=w300:dbl, "Linear"=w301:dbl)  [unwired: 4 in, 2 out]
                n223 = global read "Drive_Globals.vi" "Drive_Set_Notifier"() -> (w298:refnum<notifier>)
                n224 = Bundle By Name(cluster=T14 {"Control_State"=enum."Percent_Voltage_Control", "Angular_Throttle"=0.0, "Linear_Throttle"=0.0, "Torque_Changing"=FALSE, "Step"=0.0, "Parameter_1"=0.0, "Parameter_2"=0.0, "Parameter_3"=0.0, "Parameter_4"=0.0, "Auto_Notifier"=refnum} ("Drive_Cluster"), "Angular_Throttle"=w300, "Linear_Throttle"=w301) -> (w302:T14)
                n225 = Send Notification(notification=w302, notifier=w298) -> ()  [unwired: 1 in, 2 out]
              }
            }
            frame "No-Op", Default {
              # "Do Nothing"
            }
          }
        }
      }
    }
    frame Enabled {
    }
  }
